vi "Slow Loop Control Select.vi"(8 "Slow Loop Gain Multiplier":dbl, 9 "Commanded Slow Sample rate":dbl, 10 "Controller - User Input":T2={"Num Fast Loop"=[-11.0745, 19.702, -8.7598], "Den Fast Loop"=[1.0, -1.49756, 0.49756], "Fast Loop Gain"=1.0, "IMU_sample_rate"=0, "Num Slow Loop"=[0.1636, -0.16289, 0.0], "Den Slow Loop"=[1.0, -0.6326, 0.0], "Slow Loop Gain"=1.0, "Slow Loop sample rate"=20.0}, 11 "Controller Select":T1(ring)=enum."100hz/100hz" caption="Enum") -> (3 "Slow Loop Gains":T3)   [LabVIEW 2014]
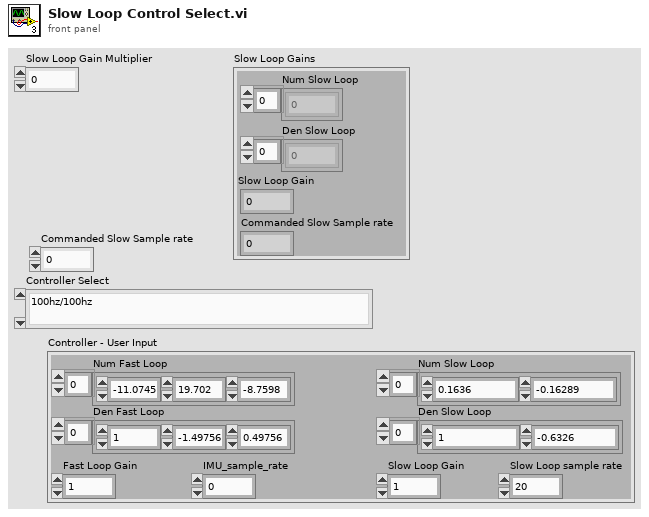
[diagram p1: front panel]
types:
  T1 = enum16{"100hz/50hz", "100hz/100hz", "200hz/200hz", "200hz/20hz", "User Defined"}
  T2 = cluster{"Num Fast Loop":dbl[], "Den Fast Loop":dbl[], "Fast Loop Gain":dbl, "IMU_sample_rate":i32, "Num Slow Loop":dbl[], "Den Slow Loop":dbl[], "Slow Loop Gain":dbl, "Slow Loop sample rate":dbl}
  T3 = cluster{"Num Slow Loop":dbl[], "Den Slow Loop":dbl[], "Slow Loop Gain":dbl, "Commanded Slow Sample rate":dbl}
  T4 = cluster{"Num Outer Loop":dbl[], "Den Outer Loop":dbl[], dbl, "Commanded Slow Sample rate":dbl}
  T5 = cluster{"Num Slow Loop":dbl[], "Den Slow Loop":dbl[], dbl, "Commanded Slow Sample rate":dbl}
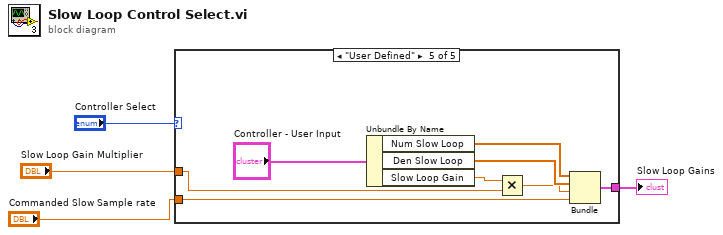
[diagram p0: block diagram]
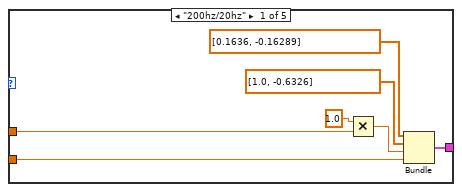
[diagram p2: hidden frame]
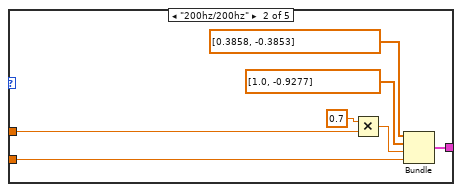
[diagram p3: hidden frame]
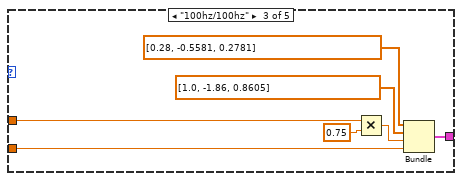
[diagram p4: hidden frame]
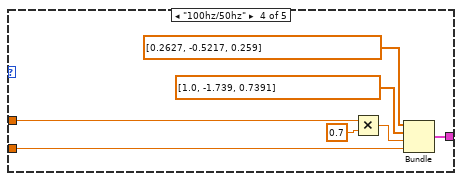
[diagram p5: hidden frame]
diagram:
  n1 = case shown="\"User Defined\"" "Controller Select" {
    tunnel: [w9 w15 w22 w29 w37] -> w3
    tunnel: "Commanded Slow Sample rate" -> [w8 w14 w21 w28 w40]
    tunnel: "Slow Loop Gain Multiplier" -> [w5 w12 w19 w26 w35]
    frame "200hz/20hz" {
      n2 = Multiply(x=1.0 ("Outer Loop Gain"), y=w5) -> (x*y=w6:dbl)
      n3 = Bundle("Num Outer Loop"=dbl[] [0.1636, -0.16289], "Den Outer Loop"=dbl[] [1.0, -0.6326], w6, "Commanded Slow Sample rate"=w8) -> (w9:T4)  [unwired: 1 in]
    }
    frame "200hz/200hz" {
      n4 = Multiply(x=0.7 ("Outer Loop Gain"), y=w12) -> (x*y=w13:dbl)
      n5 = Bundle("Num Outer Loop"=dbl[] [0.3858, -0.3853], "Den Outer Loop"=dbl[] [1.0, -0.9277], w13, "Commanded Slow Sample rate"=w14) -> (w15:T4)  [unwired: 1 in]
    }
    frame "100hz/100hz" {
      n6 = Multiply(x=w19, y=0.75 ("Outer Loop Gain")) -> (x*y=w20:dbl)
      n7 = Bundle("Num Outer Loop"=dbl[] [0.28, -0.5581, 0.2781], "Den Outer Loop"=dbl[] [1.0, -1.86, 0.8605], w20, "Commanded Slow Sample rate"=w21) -> (w22:T4)  [unwired: 1 in]
    }
    frame "100hz/50hz" {
      n8 = Multiply(x=w26, y=0.7 ("Outer Loop Gain")) -> (x*y=w27:dbl)
      n9 = Bundle("Num Outer Loop"=dbl[] [0.2627, -0.5217, 0.259], "Den Outer Loop"=dbl[] [1.0, -1.739, 0.7391], w27, "Commanded Slow Sample rate"=w28) -> (w29:T4)  [unwired: 1 in]
    }
    frame "User Defined" {
      n10 = Unbundle By Name("Controller - User Input") -> ("Num Slow Loop"=w39:dbl[], "Den Slow Loop"=w38:dbl[], "Slow Loop Gain"=w33:dbl)
      n11 = Multiply(x=w33, y=w35) -> (x*y=w34:dbl)
      n12 = Bundle("Num Slow Loop"=w39, "Den Slow Loop"=w38, w34, "Commanded Slow Sample rate"=w40) -> (w37:T5)  [unwired: 1 in]
    }
  }
  "Slow Loop Gains" <- w3
